vi "CR-CCD表面检测获取图像.vi"(7 "Session Out CCD2":T1, 8 "error in (no error)":errorcluster caption="错误输入（无错误）", 10 "Image Name":string="I1", 11 "ParamsUI":T2={"IsNorImage"=FALSE, "Exposure Values"=50000, "ImagePath"=path "C:/Users/hedongpo/Desktop/514-hdp/Alignment Assemble System/Test Picture/B/3.bmp", "相机选择"="cam4"} caption="参数界面" {"Exposure Values" scale=0.0..200000.0}) -> (0 "error out":errorcluster={"status"=TRUE, "code"=-1074360316, "source"="AMX-CCD1获取图像.vi->LabVIEW Function Structure.vi中的属性节点 (arg 1)"} caption="错误输出", 2 "Session Out":T1, 3 "Image out":T3(plugin-control), 4 "数值":dbl)   [LabVIEW 2017]
uses:
  <vilib>/userdefined/High Color/IMAQdx.ctl
  <vilib>/vision/driver/IMAQdx.llb/IMAQdx Buffer Number Mode.ctl
  <resource>/objmgr/imaqdx.rc
  Global System.vi
  <vilib>/vision/driver/NI_Vision_Acquisition_Software.lvlib
  <vilib>/vision/NI_Vision_Development_Module.lvlib
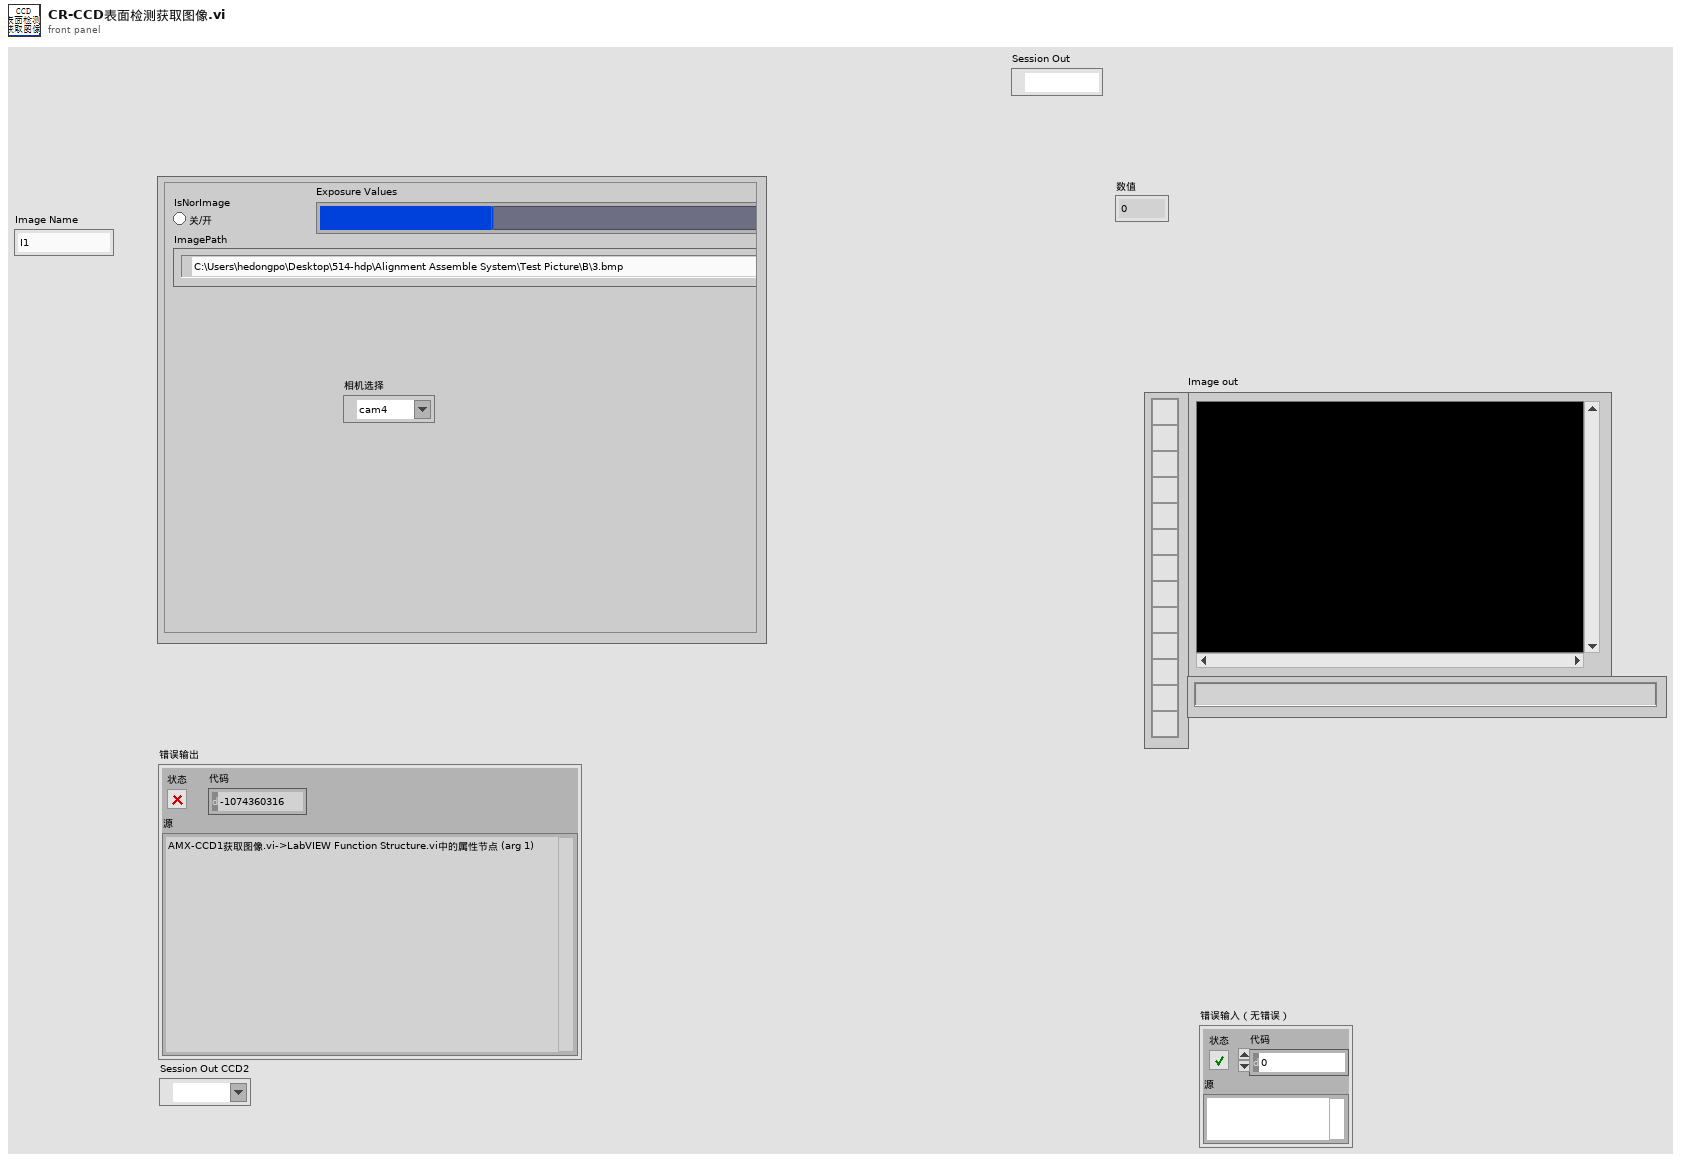
[diagram p1: front panel]
types:
  T1 = typedef "IMAQdx.ctl" = refnum<k21>
  T2 = cluster{"IsNorImage":bool, "Exposure Values":i64, "ImagePath":path, "相机选择":T1}
  T3 = typedef "IMAQ Image.ctl" = refnum<image>
  T4 = typedef "Image Type" = u32
  T5 = typedef "NI_Vision_Acquisition_Software.lvlib/IMAQdx Buffer Number Mode.ctl" = enum32{"Next", "Last", "Buffer Number", "Every", "Last New"}
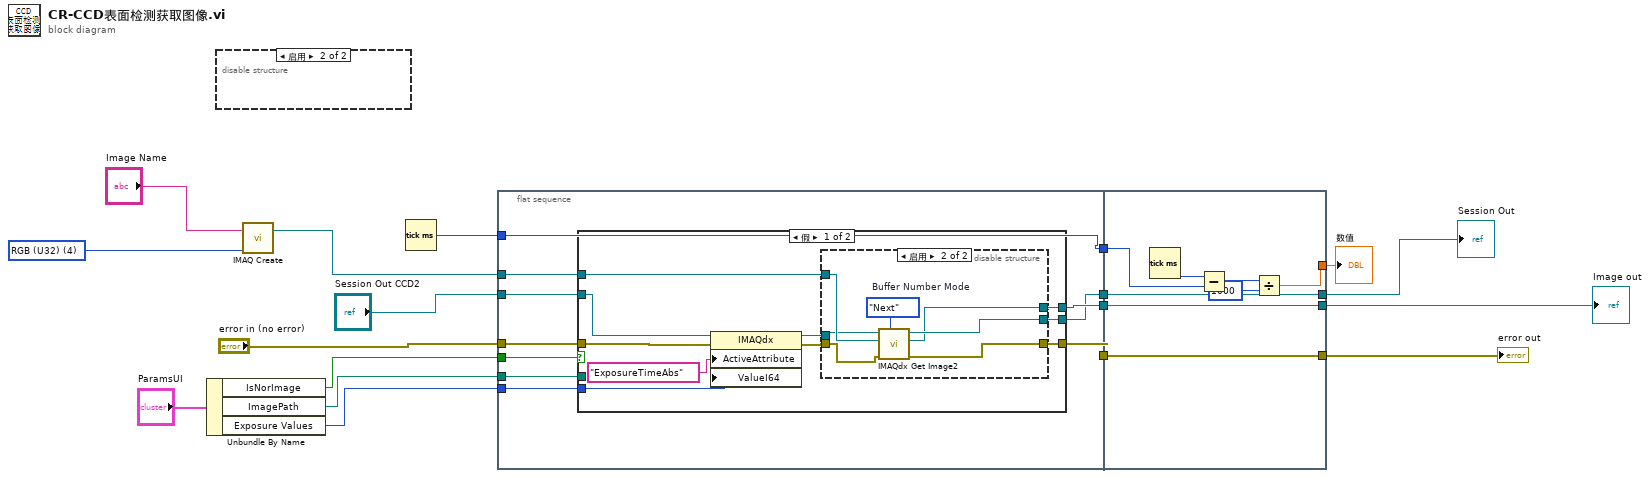
[diagram p0: block diagram]
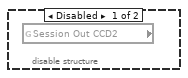
[diagram p2: hidden frame]
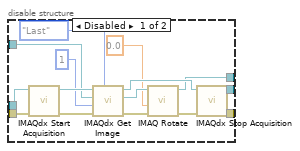
[diagram p3: hidden frame]
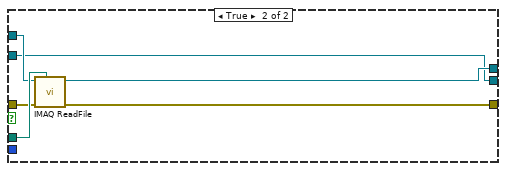
[diagram p4: hidden frame]
diagram:
  w13 = T4 4 items=["Grayscale (U8)", "Grayscale (I16)", "Grayscale (SGL)", "Complex (CSG)", "RGB (U32)", "HSL (U32)", "RGB (U64)", "Grayscale (U16)"] ("Image Type")
  n1 = Unbundle By Name("ParamsUI") -> ("IsNorImage"=w3:bool, "ImagePath"=w2:path, "Exposure Values"=w18:i64)
  n2 = disable-structure shown="启用" {
    frame Disabled {
      n3 = global read "Global System.vi" "Session Out CCD2"() -> ()  [unwired: 1 out]
    }
    frame Enabled {
    }
  }
  n4 = call "IMAQ Create"("Image Name"="Image Name", "Image Type"=w13) -> ("New Image"=w16:T3)  [unwired: 3 in, 1 out]
  n5 = Tick Count (ms)() -> (millisecond timer value=w9:u32)
  n6 = flat-sequence {
    tunnel: w3 -> [w28]
    tunnel: w2 -> [w27]
    tunnel: w18 -> [w26]
    tunnel: w16 -> [w25]
    tunnel: "error in (no error)" -> [w24]
    tunnel: "Session Out CCD2" -> [w21]
    tunnel: w9 -> [w19]
    tunnel: [w23] -> w8
    tunnel: [w22] -> w7
    tunnel: [w20] -> w6
    tunnel: [w19] -> w5
    tunnel: [w72] -> w10
    tunnel: [w73] -> w11
    tunnel: [w74] -> w14
    tunnel: w8 -> [w74]
    tunnel: w7 -> [w73]
    tunnel: w6 -> [w72]
    tunnel: w5 -> [w70]
    tunnel: [w67] -> w4
    frame #0 {
      n7 = case shown="假" w28 {
        tunnel: w27 -> [_ w66]
        tunnel: [w37 w65] -> w22
        tunnel: w26 -> [w33 _]
        tunnel: w21 -> [w29 w61]
        tunnel: w25 -> [w38 w64]
        tunnel: w24 -> [w34 w63]
        tunnel: [w35 w62] -> w23
        tunnel: [w36 w61] -> w20
        frame False {
          n8 = property class="IMAQdx"(reference=w29, error in=w34, "ActiveAttribute"="ExposureTimeAbs", "ValueI64"=w33) -> (reference out=w32:T1, error out=w31:errorcluster)
          n9 = disable-structure shown="启用" {
            disable-tunnel: w38 -> [w44 w59]
            disable-tunnel: [w43 w55] -> w37
            disable-tunnel: [w42 w56] -> w36
            disable-tunnel: [w41 w54] -> w35
            disable-tunnel: w32 -> [w40 w58]
            disable-tunnel: w31 -> [w39 w57]
            frame Disabled {
              n10 = call <vilib>:"IMAQdx Start Acquisition.vi"("error in"=w39, "Session In"=w40) -> ("error out"=w52:errorcluster, "Session Out"=w53:T1)  [unwired: 8 in]
              n11 = call <vilib>:"IMAQdx Get Image.vi"("Buffer Number Mode (Next)"=IMAQdx_Buffer_Number_Mode."Last", "error in"=w52, "Buffer Number In"=u32 1, "Image In"=w44, "Session In"=w53) -> ("error out"=w47:errorcluster, "Image Out"=w48:T3, "Session Out"=w49:T1)  [unwired: 3 in, 1 out]
              n12 = call "IMAQ Rotate"("error in (no error)"=w47, "Angle (degrees)"=sgl 0.0, "Image Src"=w48) -> ("error out"=w46:errorcluster, "Image Dst Out"=w43:T3)  [unwired: 7 in]
              n13 = call <vilib>:"IMAQdx Stop Acquisition.vi"("error in"=w46, "Session In"=w49) -> ("error out"=w41:errorcluster, "Session Out"=w42:T1)  [unwired: 8 in]
            }
            frame Enabled {
              w60 = IMAQdx_Buffer_Number_Mode."Next"  # Buffer Number Mode
              n14 = call <vilib>:"IMAQdx Get Image2.vi"("Buffer Number Mode (Next)"=w60, "error in"=w57, "Image In"=w59, "Session In"=w58) -> ("error out"=w54:errorcluster, "Image Out"=w55:T3, "Session Out"=w56:T1)  [unwired: 4 in, 1 out]
            }
          }
        }
        frame True {
          n15 = call "IMAQ ReadFile"("File Path"=w66, "error in (no error)"=w63, "Image"=w64) -> ("error out"=w62:errorcluster, "Image Out"=w65:T3)  [unwired: 4 in, 3 out]
        }
      }
    }
    frame #1 {
      n16 = Tick Count (ms)() -> (millisecond timer value=w71:u32)
      n17 = Subtract(x=w71, y=w70) -> (x-y=w69:u32)
      n18 = Divide(x=w69, y=u32 1000) -> (x/y=w67:dbl)
    }
  }
  "Image out" <- w11
  "error out" <- w14
  "Session Out" <- w10
  "数值" <- w4
